vi "Wait_nodaq_nocrio.vi"(1 "PS type":enum16{"NHR", "ITECH"}(ring), 9 "PS VISA in":refnum<visa-resource-name>, 11 "PS error in":errorcluster caption="PS error in (no error)", 12 "Wait Filepath":path=path "C:/Users/ga11/Desktop/VI/results/3PtestChrgRest.lvm" caption="Filename", 13 "Wait time":dbl) -> (10 "PS Visa Out":refnum<visa-resource-name>, 15 "PS error out":errorcluster)   [LabVIEW 2020]
uses:
  Drivers-NHR-9200/NHR/Public/Data/Read (Ave Current).vi
  Drivers-NHR-9200/NHR/Public/Data/Low Level/Fetch (Ave Voltage).vi
  Drivers-Essentials/NH Research Regenerative Test Series.lvlib
  Drivers-IT-M3400/IT-M3400.lvlib
panel:
  out "Ave Current (A)":dbl
  out "Ave Voltage (V)":dbl
  out "WaitElapsed Time (s)":i32 caption="Elapsed Time (s)"
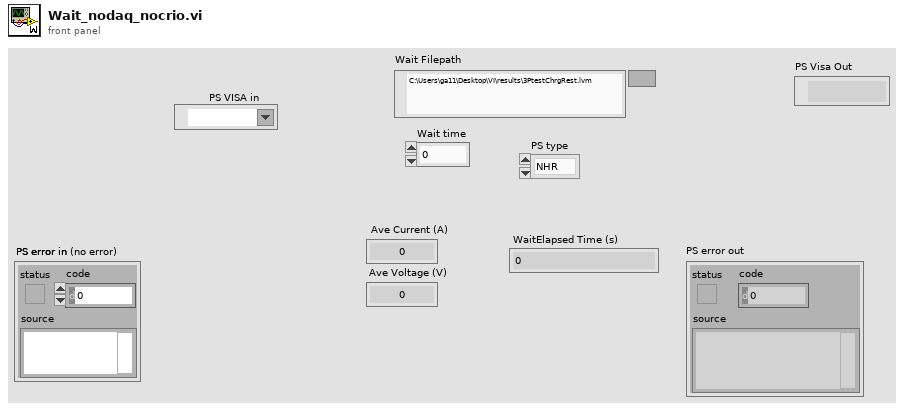
[diagram p1: front panel]
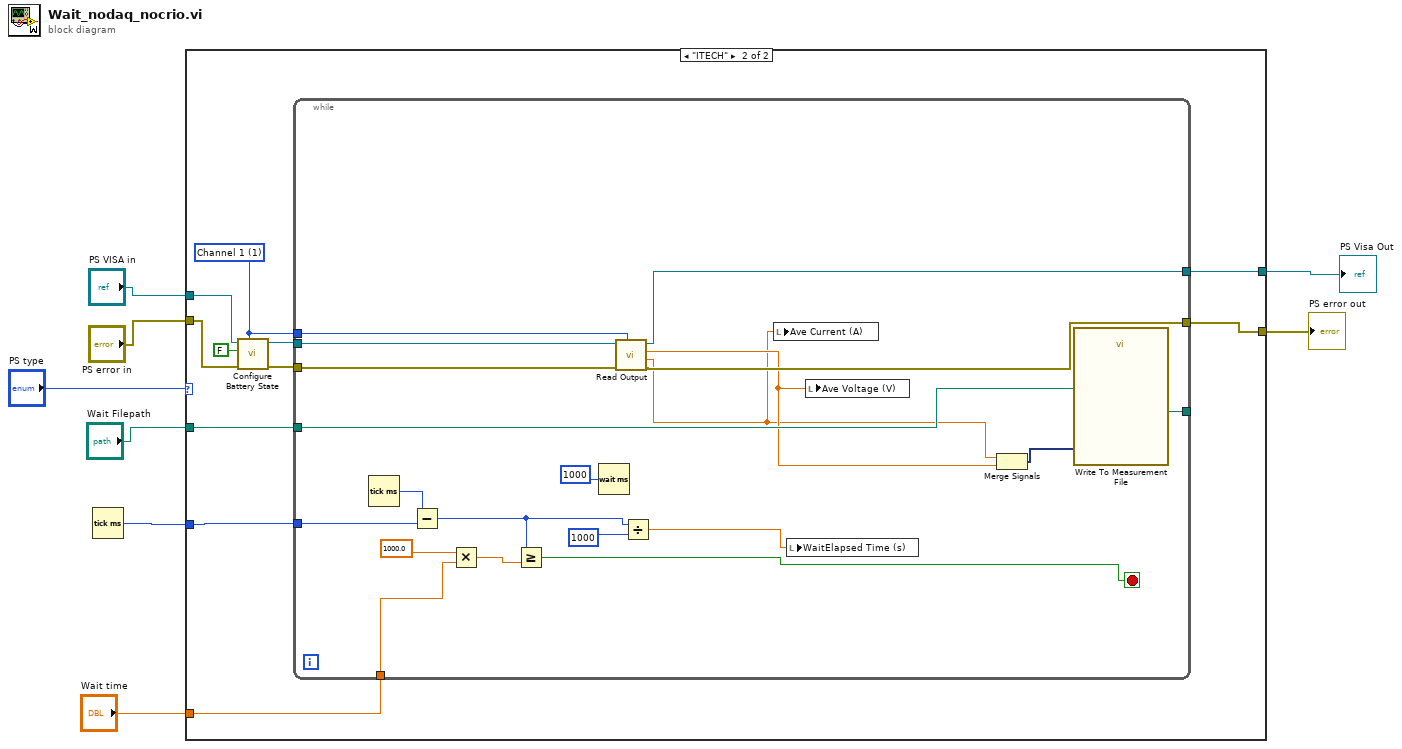
[diagram p0: block diagram]
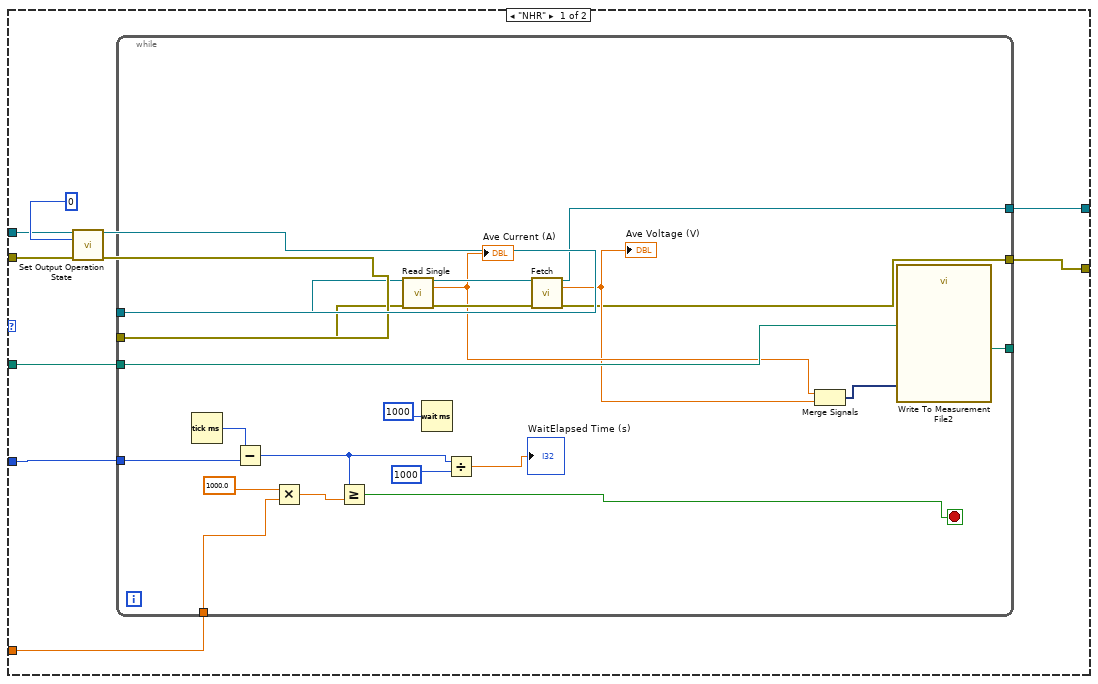
[diagram p2: hidden frame]
diagram:
  n1 = Tick Count (ms)() -> (millisecond timer value=w7:u32)
  n2 = case shown="\"ITECH\"" "PS type" {
    tunnel: "Wait time" -> [w15 w50]
    tunnel: w7 -> [w14 w49]
    tunnel: "PS VISA in" -> [w13 w43]
    tunnel: "PS error in" -> [w12 w42]
    tunnel: "Wait Filepath" -> [w11 w48]
    tunnel: [w10 w47] -> w3
    tunnel: [w9 w46] -> w2
    frame "NHR" {
      n3 = call "Set Output Operation State.vi"("VISA resource name"=w13, "Mode (0: Off)"=0, "error in (no error)"=w12) -> ("VISA resource name out"=w17:refnum<visa-resource-name>, "error out"=w16:errorcluster)  [unwired: 11 in]
      n4 = while {
        tunnel: w17 -> [w37]
        tunnel: w16 -> [w36]
        tunnel: w15 -> [w32]
        tunnel: [w29] -> _
        tunnel: w14 -> [w28]
        tunnel: w11 -> [w27]
        tunnel: [w20] -> w10
        tunnel: [w19] -> w9
        stop <- w33 stop-if-true
        n5 = Tick Count (ms)() -> (millisecond timer value=w34:u32)
        n6 = Subtract(x=w34, y=w28) -> (x-y=w26:u32)
        n7 = Multiply(x=1000.0, y=w32) -> (x*y=w30:dbl)
        n8 = Greater Or Equal?(x=w26, y=w30) -> (x >= y?=w33:bool)
        n9 = call-poly "Read Single.vi"("VISA resource name"=w37, "error in (no error)"=w36) -> ("VISA resource name out"=w38:refnum<visa-resource-name>, "Ave Current (A)"=w23:dbl, "error out"=w39:errorcluster)  [unwired: 11 in]
        "Ave Current (A)" <- w23
        n10 = Wait (ms)(milliseconds to wait=1000) -> ()  [unwired: 1 out]
        n11 = Divide(x=w26, y=1000) -> (x/y=→"WaitElapsed Time (s)":dbl)
        n12 = call-poly "Fetch.vi"("VISA resource name"=w38, "error in (no error)"=w39) -> ("VISA resource name out"=w20:refnum<visa-resource-name>, "Ave Voltage (V)"=w21:dbl, "error out"=w19:errorcluster)  [unwired: 11 in]
        "Ave Voltage (V)" <- w21
        n13 = Merge Signals "Merge Signals"(w23, w21) -> (w22:dynamicdata)
        n14 = call "Write To Measurement File2"("Signals"=w22, "Filename"=w27) -> ("Filename Out"=w29:path)  [unwired: 15 in, 2 out]
      }
    }
    frame "ITECH" {
      w40 = 1 items=["Channel 1"=1, "Channel 2"=2, "Channel 3"=3, "Channel 4"=4, "Channel 5"=5, "Channel 6"=6, "Channel 7"=7, "Channel 8"=8, "Channel 8"=9, "Channel 10"=10, "Channel 11"=11, "Channel 12"=12, "Channel 13"=13, "Channel 14"=14, "Channel 15"=15, "Channel 16"=16] ("Channel")
      n15 = call "Configure Battery State.vi"("Channel"=w40, "error in"=w42, "State"=FALSE, "VISA resource name"=w43) -> ("error out"=w44:errorcluster, "VISA resource name out"=w45:refnum<visa-resource-name>)  [unwired: 6 in]
      n16 = while {
        tunnel: w50 -> [w67]
        tunnel: [w64] -> _
        tunnel: w49 -> [w63]
        tunnel: w48 -> [w62]
        tunnel: [w58] -> w47
        tunnel: [w57] -> w46
        tunnel: w45 -> [w53]
        tunnel: w44 -> [w52]
        tunnel: w40 -> [w51]
        stop <- w68 stop-if-true
        n17 = Tick Count (ms)() -> (millisecond timer value=w69:u32)
        n18 = Subtract(x=w69, y=w63) -> (x-y=w61:u32)
        n19 = Multiply(x=1000.0, y=w67) -> (x*y=w65:dbl)
        n20 = Greater Or Equal?(x=w61, y=w65) -> (x >= y?=w68:bool)
        n21 = Wait (ms)(milliseconds to wait=1000) -> ()  [unwired: 1 out]
        n22 = call "Read Output.vi"("Channel"=w51, "error in"=w52, "VISA resource name"=w53) -> ("error out"=w57:errorcluster, "Read Current(A)"=w55:dbl, "Read Voltage(V)"=w56:dbl, "VISA resource name out"=w58:refnum<visa-resource-name>)  [unwired: 5 in]
        n23 = Divide(x=w61, y=1000) -> (x/y=w54:dbl)
        n24 = local write "Ave Current (A)"(w55) -> ()
        n25 = local write "WaitElapsed Time (s)"(w54) -> ()
        n26 = local write "Ave Voltage (V)"(w56) -> ()
        n27 = Merge Signals "Merge Signals"(w55, w56) -> (w59:dynamicdata)
        n28 = call "Write To Measurement File"("Signals"=w59, "Filename"=w62) -> ("Filename Out"=w64:path)  [unwired: 15 in, 2 out]
      }
    }
  }
  "PS Visa Out" <- w3
  "PS error out" <- w2
